vi "CMD_Wrist.vi"(1 "Line":string) -> (0 "Done":bool)   [LabVIEW 2017, in "Apple script.lvlib"]
uses:
  Apple script.lvlib
  Robot Global Data.vi
panel:
  in  "Parameters":i32[](array[numeric])=[1]
  in  "Subcommands":string[](array[string])=["to"]
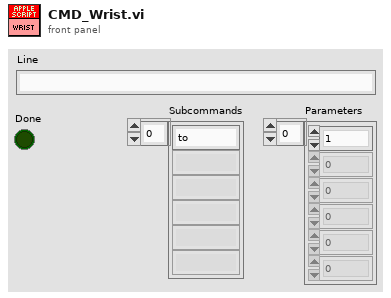
[diagram p1: front panel]
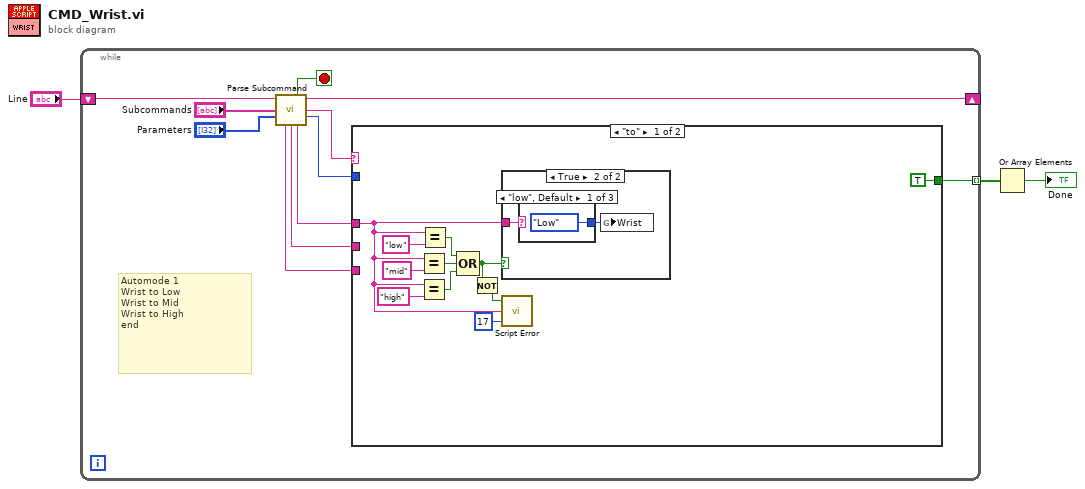
[diagram p0: block diagram]
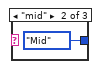
[diagram p3: hidden frame]
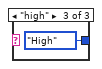
[diagram p4: hidden frame]
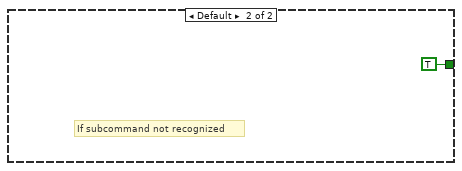
[diagram p5: hidden frame]
diagram:
  n1 = while {
    shift-right: [w11] -> _
    shift-left: "Line" -> [w14]
    tunnel: [w4] -> w2 mode=indexing
    stop <- w10 stop-if-true
    # "Automode 1\nWrist to Low\nWrist to Mid\nWrist to High\nend"
    n2 = call "Parse Subcommand.vi"("Text In"=w14, "Subcommands"="Subcommands", "Parameters"="Parameters") -> ("Done"=w10:bool, "Text Out"=w11:string, "Subcommand"=w9:string, "# of Parameters"=w8:i32, "Parameter 3"=w5:string, "Parameter 2"=w6:string, "Parameter 1"=w7:string)  [unwired: 6 in]
    n3 = case shown="\"to\"" w9 {
      tunnel: w8 -> [_ _]
      tunnel: w7 -> [w16 _]
      tunnel: w6 -> [_ _]
      tunnel: w5 -> [_ _]
      tunnel: [TRUE TRUE] -> w4
      frame "to" {
        n4 = Equal?(x=w16, y="mid") -> (x = y?=w20:bool)
        n5 = Equal?(x=w16, y="high") -> (x = y?=w19:bool)
        n6 = Equal?(x=w16, y="low") -> (x = y?=w21:bool)
        n7 = Compound Arithmetic op=OR(w21, w20, w19) -> (w18:bool)
        n8 = Not(x=w18) -> (.not. x?=w15:bool)
        n9 = case shown="True" w18 {
          tunnel: w16 -> [_ w27]
          frame False {
          }
          frame True {
            n10 = case shown="\"low\", Default" w27 {
              tunnel: [enum16{"Low", "Mid", "High"}."Low" ("Lift") enum16{"Low", "Mid", "High"}."Mid" ("Lift") enum16{"Low", "Mid", "High"}."High" ("Lift")] -> w26
              frame "low", Default {
              }
              frame "mid" {
              }
              frame "high" {
              }
            }
            n11 = global write "Robot Global Data.vi" "Wrist"(w26) -> ()
          }
        }
        n12 = call "Script Error.vi"("Error?"=w15, "Error Details"=w16, "Error Code"=17) -> ()  [unwired: 2 in, 1 out]
      }
      frame Default {
        # "If subcommand not recognized"
      }
    }
  }
  n13 = Or Array Elements(Boolean array=w2) -> (logical OR=→"Done":bool)
